vi "write_params.vi"(8 "error in (no error)":errorcluster, 10 "params":T1={"radius"=1.0, "weights"="uniform", "algorithm"="auto", "leaf_size"=30.0, "p"=2.0, "metric"="minkowski", "n_jobs"=1.0}, 11 "RadiusNeighborsRegressor in":refnum<class "RadiusNeighborsRegressor.lvclass">) -> (0 "error out":errorcluster, 3 "RadiusNeighborsRegressor out":refnum<class "RadiusNeighborsRegressor.lvclass">)   [LabVIEW 2020, in "RadiusNeighborsRegressor.lvclass"]
uses:
  RadiusNeighborsRegressor.lvclass
  Controls/radius_neighbors_regressor_params.ctl
  RadiusNeighborsRegressor.lvclass/RadiusNeighborsRegressor.ctl
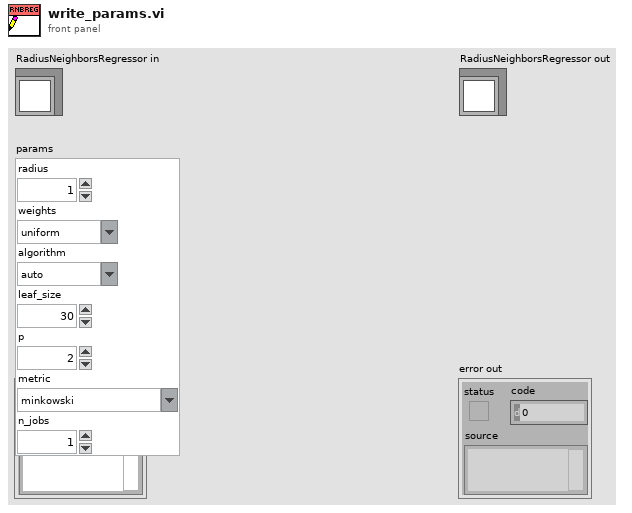
[diagram p1: front panel]
types:
  T1 = typedef "radius_neighbors_regressor_params.ctl" = cluster{"radius":dbl, "weights":string, "algorithm":string, "leaf_size":dbl, "p":dbl, "metric":string, "n_jobs":dbl}
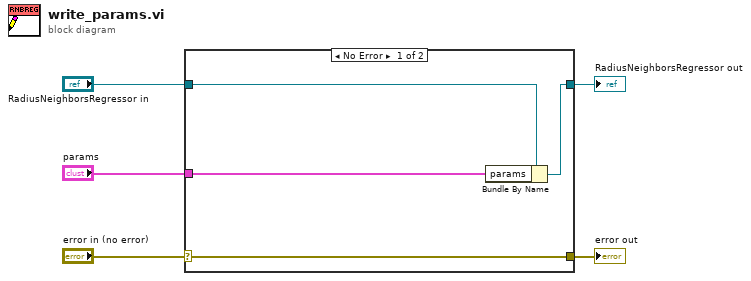
[diagram p0: block diagram]
diagram:
  n1 = case shown="No Error" "error in (no error)" {
    selector: "error in (no error)" -> [w9 w10]
    tunnel: [w9 w10] -> w4
    tunnel: [w7 w11] -> w2
    tunnel: "RadiusNeighborsRegressor in" -> [w8 w11]
    tunnel: "params" -> [w6 _]
    frame No Error {
      n2 = Bundle By Name(cluster=w8, "params"=w6) -> (w7:refnum<class "RadiusNeighborsRegressor.lvclass">)
    }
    frame Error {
    }
  }
  "error out" <- w4
  "RadiusNeighborsRegressor out" <- w2
